vi "Analyze.vi"(8 "error in (no error)":errorcluster, 10 "Image in":T1, 11 "Analyze FF Spectrum in":refnum<class "Analyze FF Spectrum.lvclass">) -> (0 "error out":errorcluster, 1 "Result":refnum<class "Analyze Results Base.lvclass">, 2 "Image out":T1, 3 "Analyze FF Spectrum out":refnum<class "Analyze FF Spectrum.lvclass">)   [LabVIEW 2014, in "Analyze.lvlib" / "Analyze FF Spectrum.lvclass"]
uses:
  Analyze FF Spectrum.lvclass
  <vilib>/vision/Image Controls.llb/IMAQ Image.ctl
  Results and Overlays/Results Base/Analyze Results Base.lvclass
  Results and Overlays/Results SRFF/Analyze Results FF-Spectrum.lvclass
  Analyze Parameter/Analyze Parameter Spectral Calibration/Analyze Parameter Spectral Calibration.lvclass
  Results and Overlays/Results SRFF/Analyze Results FF-Spectrum.lvclass/Analyze Results FF-Spectrum.ctl
  Results and Overlays/Results SRFF/Write SRFF Spectrum.vi
  Analyze BaseClass/Analyze BaseClass/Analyze BaseClass.lvclass
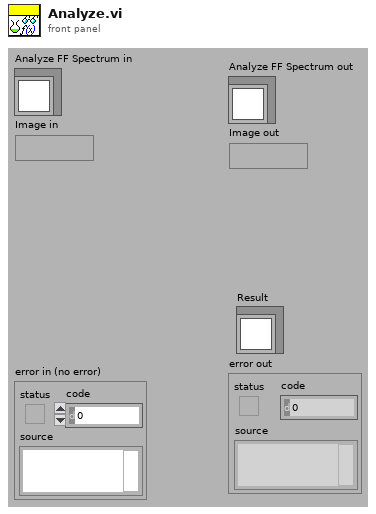
[diagram p1: front panel]
types:
  T1 = typedef "IMAQ Image.ctl" = refnum<image>
  T2 = typedef "ROI Descriptor" = cluster{"Global Rectangle":i32[], "Contours":cluster{"ID":enum32{"External", "Internal"}, "Type":u32, "Coordinates":i32[]}[]}
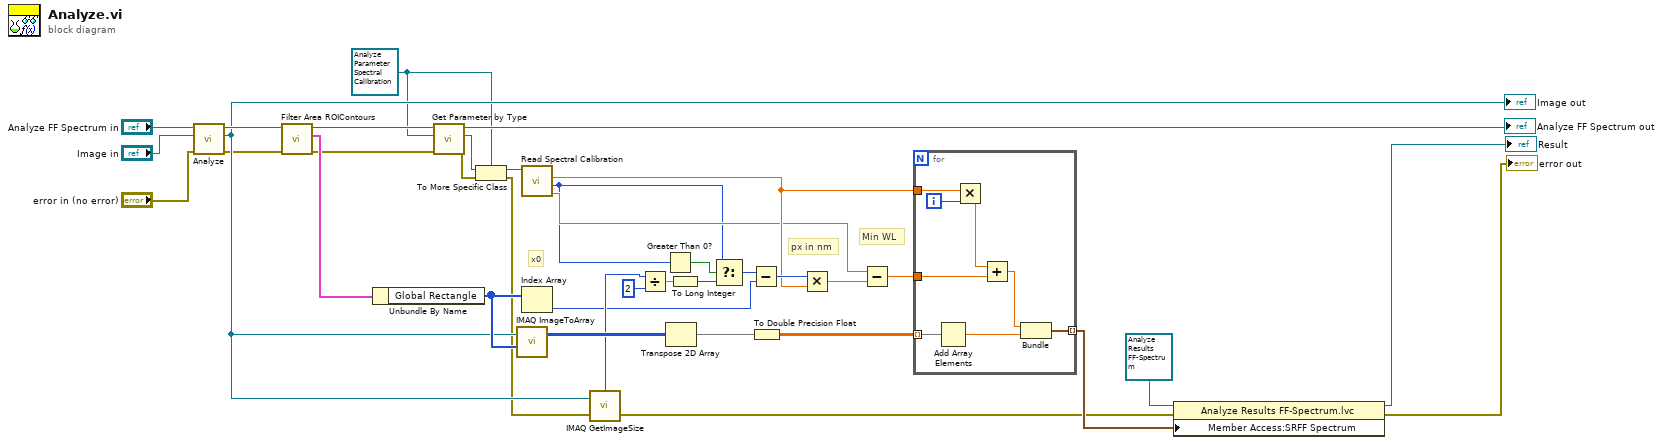
[diagram p0: block diagram]
diagram:
  w5 = refnum<class "Analyze Parameter Spectral Calibration.lvclass"> refnum ("Spectral Calibration")
  # "px in nm"
  # "x0"
  # "Min WL"
  n1 = call-parent "Analyze.vi"("error in (no error)"="error in (no error)", "Image in"="Image in", "Analyze BaseClass in"="Analyze FF Spectrum in") -> ("error out"=w20:errorcluster, "Image out"=w23:T1, "Analyze BaseClass out"=w24:refnum<class "Analyze FF Spectrum.lvclass">)  [unwired: 5 in, 1 out]
  "Image out" <- w23
  n2 = call-dynamic "Filter Area ROIContours.vi"("error in (no error)"=w20, "Analyze BaseClass in"=w24) -> ("error out"=w2:errorcluster, "ROI of Area type"=w37:T2, "Analyze BaseClass out"=w8:refnum<class "Analyze FF Spectrum.lvclass">)  [unwired: 7 in]
  n3 = Unbundle By Name(w37) -> ("Global Rectangle"=w31:i32[])
  n4 = call "Get Parameter by Type.vi"("error in (no error)"=w2, "Parameter Type"=w5, "Analyze BaseClass in"=w8) -> ("error out"=w3:errorcluster, "Parameter"=w4:refnum<class "Analyze Parameter Base.lvclass">, "Analyze BaseClass out"=→"Analyze FF Spectrum out":refnum<class "Analyze FF Spectrum.lvclass">)  [unwired: 5 in, 1 out]
  n5 = To More Specific Class(target class=w5, reference=w4, error in=w3) -> (specific class reference=w6:refnum<class "Analyze Parameter Spectral Calibration.lvclass">, error out=w1:errorcluster)
  n6 = call "IMAQ ImageToArray"("Optional Rectangle"=w31, "Image"=w23) -> ("Image Pixels (I16)"=w36:i16[][])  [unwired: 2 in, 4 out]
  n7 = call "Read Spectral Calibration.vi"("Analyze Parameter Spectral Calibration in"=w6) -> ("Central WL"=w17:dbl[unit], "Central Pixel"=w15:i32, "nm per px"=w18:dbl[unit])  [unwired: 7 in, 1 out]
  n8 = Index Array(array=w31) -> (element=w30:i32)  [unwired: 1 in]
  n9 = call "IMAQ GetImageSize"("Image"=w23, "error in (no error)"=w1) -> ("X Resolution"=w33:i32, "error out"=w12:errorcluster)  [unwired: 2 in, 1 out]
  n10 = Divide(x=w33, y=2) -> (x/y=w14:dbl)
  n11 = Greater Than 0?(x=w15) -> (x > 0?=w16:bool)
  n12 = Transpose 2D Array(2D array=w36) -> (transposed array=w34:i16[][])
  n13 = To Long Integer(number=w14) -> (32bit integer=w11:i32)
  n14 = Select(t=w15, s=w16, f=w11) -> (s? t:f=w13:i32)
  n15 = Subtract(x=w13, y=w30) -> (x-y=w29:i32)
  n16 = To Double Precision Float(number=w34) -> (double precision float=w35:dbl[][])
  n17 = Multiply(x=w29, y=w18) -> (x*y=w28:dbl[unit])
  n18 = Subtract(x=w17, y=w28) -> (x-y=w27:dbl[unit])
  n19 = for {
    tunnel: w35 -> [w45] mode=indexing
    tunnel: w27 -> [w41]
    tunnel: w18 -> [w43]
    tunnel: [w38] -> w21 mode=indexing
    i -> [w44]
    n20 = Add Array Elements(numeric array=w45) -> (sum=w39:dbl)
    n21 = Multiply(x=w43, y=w44) -> (x*y=w42:dbl[unit])
    n22 = Add(x=w42, y=w41) -> (x+y=w40:dbl[unit])
    n23 = Bundle(w40, w39) -> (w38:cluster{dbl[unit], dbl})  [unwired: 1 in]
  }
  n24 = property class="Analyze Results FF-Spectrum.lvc"(reference=refnum<class "Analyze Results FF-Spectrum.lvclass"> refnum ("Analyze Results FF-Spectrum.lvclass"), error in=w12, "Member Access:SRFF Spectrum"=w21) -> (reference out=→"Result":refnum<class "Analyze Results FF-Spectrum.lvclass">, error out=→"error out":errorcluster)
